vi "Y[i]=Clip{X[i]}.vi"(2 "lower limit":dbl format="%.2f", 3 "upper limit":dbl format="%.2f", 4 "Input Array":dbl[](array[numeric])) -> (0 "error":i32, 1 "Clipped Array":dbl[](array[numeric]))   [LabVIEW 2020, in "NI_AALPro.lvlib"]
doc: "Clips the elements of <B>Input Array</B> to within the bounds specified by <B>upper limit</B> and <B>lower limit</B>."
uses:
  <vilib>/Analysis/NI_AALPro.lvlib
panel:
  # "Y[i]=Clip{X[i]}"
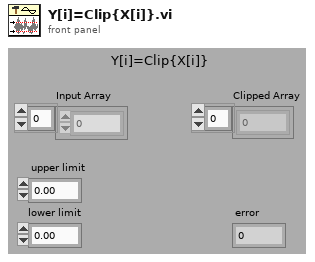
[diagram p1: front panel]
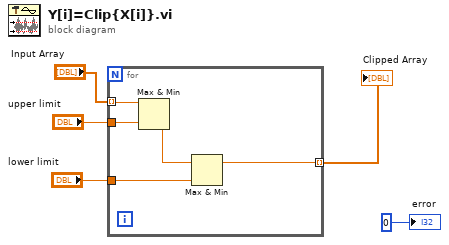
[diagram p0: block diagram]
diagram:
  n1 = for {
    tunnel: "Input Array" -> [w10] mode=indexing
    tunnel: "upper limit" -> [w9]
    tunnel: "lower limit" -> [w7]
    tunnel: [w6] -> w1 mode=indexing
    n2 = Max & Min(x=w10, y=w9) -> (min(x,y)=w8:dbl)  [unwired: 1 out]
    n3 = Max & Min(x=w8, y=w7) -> (max(x,y)=w6:dbl)  [unwired: 1 out]
  }
  "Clipped Array" <- w1
  "error" <- 0
